vi "createChannel.vi"(8 "error in (no error)":errorcluster, 11 "niDAQmxAO in":refnum<class "niDAQmxAO.lvclass">) -> (0 "error out":errorcluster, 3 "niDAQmxAO out":refnum<class "niDAQmxAO.lvclass">)   [LabVIEW 2009, in "Hardware.lvlib" / "Channels.lvlib" / "niDAQmxAO.lvclass"]
uses:
  niDAQmxAO.lvclass
  <vilib>/DAQmx/create/channels.llb/DAQmx Create Channel (AO-Voltage-Basic).vi
  niDAQmxAO.lvclass/niDAQmxAO.ctl
  <vilib>/DAQmx/create/channels.llb/DAQmx Create Channel (AO-Current-Basic).vi
  <vilib>/DAQmx/create/channels.llb/DAQmx Create Channel (AO-FuncGen).vi
  AnalogOutput.lvclass
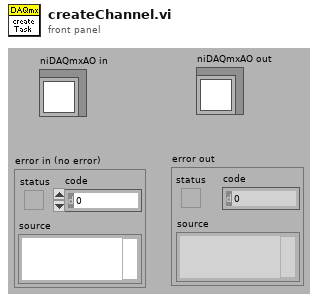
[diagram p1: front panel]
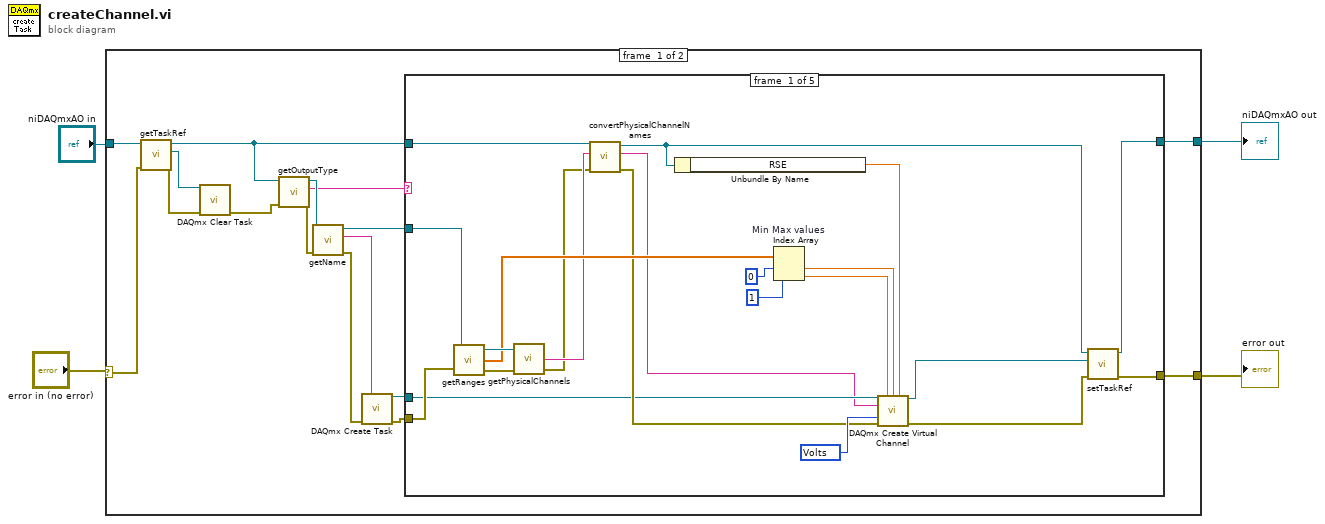
[diagram p0: block diagram]
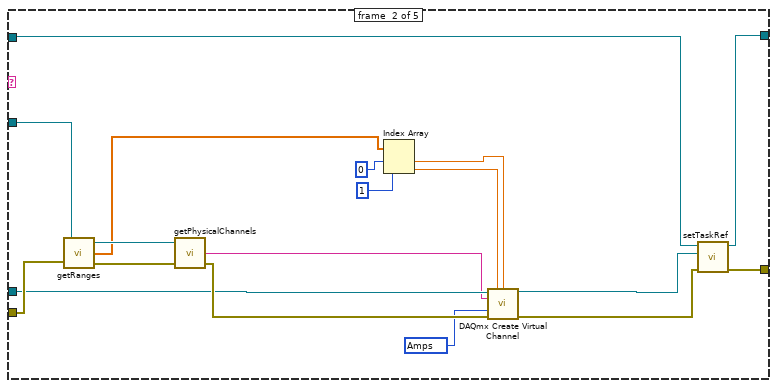
[diagram p2: hidden frame]
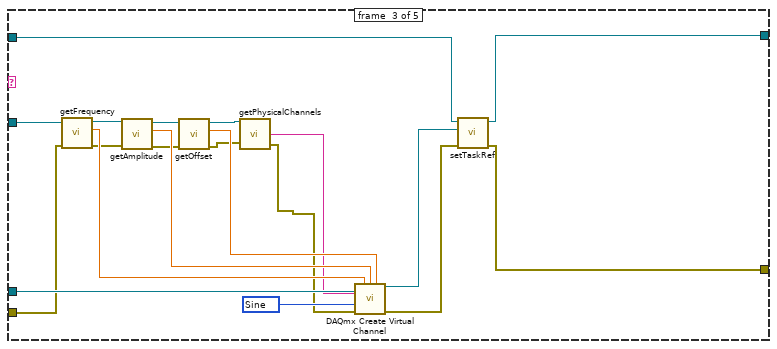
[diagram p3: hidden frame]
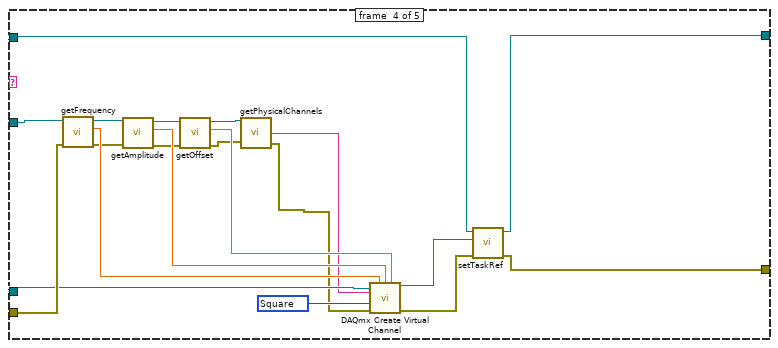
[diagram p4: hidden frame]
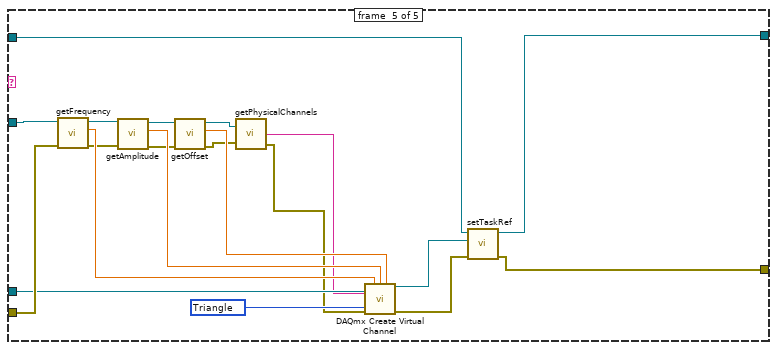
[diagram p5: hidden frame]
diagram:
  n1 = case shown="No Error" "error in (no error)" {
    selector: "error in (no error)" -> [w6 w121]
    tunnel: "niDAQmxAO in" -> [w10 w122]
    tunnel: [w20 w121] -> w2
    tunnel: [w19 w122] -> w1
    frame #0 {
      n2 = call "getTaskRef.vi"("error in (no error)"=w6, "niDAQmxAO.lvclass in"=w10) -> ("error out"=w7:errorcluster, "DAQmx Task Ref"=w8:refnum<k21>, "niDAQmxAO.lvclass out"=w9:refnum<class "niDAQmxAO.lvclass">)  [unwired: 7 in]
      n3 = call <vilib>:"DAQmx Clear Task.vi"("task in"=w8, "error in"=w7) -> ("error out"=w5:errorcluster)  [unwired: 13 in]
      n4 = call "getOutputType.vi"("error in (no error)"=w5, "AnalogOutput.lvclass in"=w9) -> ("error out"=w16:errorcluster, "Output Type"=w15:string, "AnalogOutput.lvclass out"=w17:refnum<class "niDAQmxAO.lvclass">)  [unwired: 7 in]
      n5 = call "getName.vi"("error in (no error)"=w16, "AnalogOutput.lvclass in"=w17) -> ("error out"=w12:errorcluster, "name"=w11:string, "AnalogOutput.lvclass out"=w18:refnum<class "niDAQmxAO.lvclass">)  [unwired: 7 in]
      n6 = call <vilib>:"DAQmx Create Task.vi"("new task name"=w11, "error in"=w12) -> ("task out"=w14:refnum<k21>, "error out"=w13:errorcluster)  [unwired: 12 in]
      n7 = case shown="\"Voltage\", Default" w15 {
        tunnel: w18 -> [w41 w53 w77 w87 w107]
        tunnel: w14 -> [w22 w51 w66 w85 w105]
        tunnel: w13 -> [w40 w52 w65 w86 w106]
        tunnel: w9 -> [w27 w50 w68 w88 w108]
        tunnel: [w37 w54 w63 w83 w103] -> w20
        tunnel: [w36 w55 w64 w84 w104] -> w19
        frame #0 {
          w29 = u16 10348 items=["Volts"=10348]
          n8 = call "getRanges.vi"("AnalogOutput.lvclass in"=w41, "error in (no error)"=w40) -> ("AnalogOutput.lvclass out"=w35:refnum<class "niDAQmxAO.lvclass">, "Ranges"=w28:dbl[], "error out"=w34:errorcluster)
          n9 = call-dynamic "getPhysicalChannels.vi"("AnalogOutput.lvclass in"=w35, "error in (no error)"=w34) -> ("Physical Channels"=w25:string, "error out"=w24:errorcluster)  [unwired: 1 out]
          n10 = call "convertPhysicalChannelNames.vi"("error in (no error)"=w24, "PhysicalChannels"=w25, "niDAQmxAO.lvclass in"=w27) -> ("error out"=w23:errorcluster, "channel_names"=w21:string, "niDAQmxAO.lvclass out"=w26:refnum<class "niDAQmxAO.lvclass">)  [unwired: 6 in]
          n11 = Unbundle By Name(w26) -> ("RSE"=w42:dbl)
          n12 = Index Array "Min Max values"(array=w28, index #1=0, index #2=1) -> (element #1=w31:dbl, element #2=w30:dbl)
          n13 = call-poly <vilib>:"DAQmx Create Virtual Channel.vi"("task in"=w22, "maximum value"=w30, "minimum value"=w31, "output terminal configuration"=w42, "physical channels"=w21, "units"=w29, "error in"=w23) -> ("task out"=w39:refnum<k21>, "error out"=w38:errorcluster)  [unwired: 7 in]
          n14 = call "setTaskRef.vi"("error in (no error)"=w38, "DAQmx Task Ref"=w39, "niDAQmxAO.lvclass in"=w26) -> ("error out"=w37:errorcluster, "niDAQmxAO.lvclass out"=w36:refnum<class "niDAQmxAO.lvclass">)  [unwired: 7 in]
        }
        frame #1 {
          w47 = u16 10342 items=["Amps"=10342]
          n15 = call "getRanges.vi"("AnalogOutput.lvclass in"=w53, "error in (no error)"=w52) -> ("AnalogOutput.lvclass out"=w58:refnum<class "niDAQmxAO.lvclass">, "Ranges"=w46:dbl[], "error out"=w59:errorcluster)
          n16 = call-dynamic "getPhysicalChannels.vi"("AnalogOutput.lvclass in"=w58, "error in (no error)"=w59) -> ("Physical Channels"=w43:string, "error out"=w60:errorcluster)  [unwired: 1 out]
          n17 = Index Array(array=w46, index #1=0, index #2=1) -> (element #1=w44:dbl, element #2=w45:dbl)
          n18 = call-poly <vilib>:"DAQmx Create Virtual Channel.vi"("task in"=w51, "maximum value"=w45, "minimum value"=w44, "physical channels"=w43, "units"=w47, "error in"=w60) -> ("task out"=w56:refnum<k21>, "error out"=w57:errorcluster)  [unwired: 8 in]
          n19 = call "setTaskRef.vi"("error in (no error)"=w57, "DAQmx Task Ref"=w56, "niDAQmxAO.lvclass in"=w50) -> ("error out"=w54:errorcluster, "niDAQmxAO.lvclass out"=w55:refnum<class "niDAQmxAO.lvclass">)  [unwired: 7 in]
        }
        frame #2 {
          w67 = u16 14751 items=["Sine"=14751]
          n20 = call "getFrequency.vi"("error in (no error)"=w65, "AnalogOutput.lvclass in"=w77) -> ("error out"=w74:errorcluster, "Frequency"=w76:dbl, "AnalogOutput.lvclass out"=w75:refnum<class "niDAQmxAO.lvclass">)  [unwired: 7 in]
          n21 = call "getAmplitude.vi"("error in (no error)"=w74, "AnalogOutput.lvclass in"=w75) -> ("error out"=w72:errorcluster, "Amplitude"=w73:dbl, "AnalogOutput.lvclass out"=w71:refnum<class "niDAQmxAO.lvclass">)  [unwired: 7 in]
          n22 = call "getOffset.vi"("error in (no error)"=w72, "AnalogOutput.lvclass in"=w71) -> ("error out"=w69:errorcluster, "Offset"=w78:dbl, "AnalogOutput.lvclass out"=w70:refnum<class "niDAQmxAO.lvclass">)  [unwired: 7 in]
          n23 = call-dynamic "getPhysicalChannels.vi"("AnalogOutput.lvclass in"=w70, "error in (no error)"=w69) -> ("Physical Channels"=w62:string, "error out"=w61:errorcluster)  [unwired: 1 out]
          n24 = call-poly <vilib>:"DAQmx Create Virtual Channel.vi"("task in"=w66, "frequency"=w76, "amplitude"=w73, "offset"=w78, "physical channels"=w62, "type"=w67, "error in"=w61) -> ("task out"=w79:refnum<k21>, "error out"=w80:errorcluster)  [unwired: 7 in]
          n25 = call "setTaskRef.vi"("error in (no error)"=w80, "DAQmx Task Ref"=w79, "niDAQmxAO.lvclass in"=w68) -> ("error out"=w63:errorcluster, "niDAQmxAO.lvclass out"=w64:refnum<class "niDAQmxAO.lvclass">)  [unwired: 7 in]
        }
        frame #3 {
          w89 = u16 14753 items=["Square"=14753]
          n26 = call "getFrequency.vi"("error in (no error)"=w86, "AnalogOutput.lvclass in"=w87) -> ("error out"=w95:errorcluster, "Frequency"=w97:dbl, "AnalogOutput.lvclass out"=w96:refnum<class "niDAQmxAO.lvclass">)  [unwired: 7 in]
          n27 = call "getAmplitude.vi"("error in (no error)"=w95, "AnalogOutput.lvclass in"=w96) -> ("error out"=w93:errorcluster, "Amplitude"=w94:dbl, "AnalogOutput.lvclass out"=w92:refnum<class "niDAQmxAO.lvclass">)  [unwired: 7 in]
          n28 = call "getOffset.vi"("error in (no error)"=w93, "AnalogOutput.lvclass in"=w92) -> ("error out"=w90:errorcluster, "Offset"=w98:dbl, "AnalogOutput.lvclass out"=w91:refnum<class "niDAQmxAO.lvclass">)  [unwired: 7 in]
          n29 = call-dynamic "getPhysicalChannels.vi"("AnalogOutput.lvclass in"=w91, "error in (no error)"=w90) -> ("Physical Channels"=w82:string, "error out"=w81:errorcluster)  [unwired: 1 out]
          n30 = call-poly <vilib>:"DAQmx Create Virtual Channel.vi"("task in"=w85, "frequency"=w97, "amplitude"=w94, "offset"=w98, "physical channels"=w82, "type"=w89, "error in"=w81) -> ("task out"=w99:refnum<k21>, "error out"=w100:errorcluster)  [unwired: 7 in]
          n31 = call "setTaskRef.vi"("error in (no error)"=w100, "DAQmx Task Ref"=w99, "niDAQmxAO.lvclass in"=w88) -> ("error out"=w83:errorcluster, "niDAQmxAO.lvclass out"=w84:refnum<class "niDAQmxAO.lvclass">)  [unwired: 7 in]
        }
        frame #4 {
          w109 = u16 14752 items=["Triangle"=14752]
          n32 = call "getFrequency.vi"("error in (no error)"=w106, "AnalogOutput.lvclass in"=w107) -> ("error out"=w115:errorcluster, "Frequency"=w117:dbl, "AnalogOutput.lvclass out"=w116:refnum<class "niDAQmxAO.lvclass">)  [unwired: 7 in]
          n33 = call "getAmplitude.vi"("error in (no error)"=w115, "AnalogOutput.lvclass in"=w116) -> ("error out"=w113:errorcluster, "Amplitude"=w114:dbl, "AnalogOutput.lvclass out"=w112:refnum<class "niDAQmxAO.lvclass">)  [unwired: 7 in]
          n34 = call "getOffset.vi"("error in (no error)"=w113, "AnalogOutput.lvclass in"=w112) -> ("error out"=w110:errorcluster, "Offset"=w118:dbl, "AnalogOutput.lvclass out"=w111:refnum<class "niDAQmxAO.lvclass">)  [unwired: 7 in]
          n35 = call-dynamic "getPhysicalChannels.vi"("AnalogOutput.lvclass in"=w111, "error in (no error)"=w110) -> ("Physical Channels"=w102:string, "error out"=w101:errorcluster)  [unwired: 1 out]
          n36 = call-poly <vilib>:"DAQmx Create Virtual Channel.vi"("task in"=w105, "frequency"=w117, "amplitude"=w114, "offset"=w118, "physical channels"=w102, "type"=w109, "error in"=w101) -> ("task out"=w119:refnum<k21>, "error out"=w120:errorcluster)  [unwired: 7 in]
          n37 = call "setTaskRef.vi"("error in (no error)"=w120, "DAQmx Task Ref"=w119, "niDAQmxAO.lvclass in"=w108) -> ("error out"=w103:errorcluster, "niDAQmxAO.lvclass out"=w104:refnum<class "niDAQmxAO.lvclass">)  [unwired: 7 in]
        }
      }
    }
    frame #1 {
    }
  }
  "error out" <- w2
  "niDAQmxAO out" <- w1
